vi "SDKSID4_Array Analysis.vi"(0 "SDKSID4 session In":T1, 1 "Interferogram in (ArrayI16)":i16[][](array[numeric]), 11 "error in (no error)":errorcluster) -> (4 "SDKSID4 session Out":T1, 6 "Intensity out":sgl[][](array[numeric]), 10 "Phase out":sgl[][](array[numeric]), 14 "Tilt information out":cluster{"X-tilt":sgl, "Y-tilt":sgl}, 15 "error out":errorcluster)   [LabVIEW 2013]
doc: "This VI analyses an input interferogram (a 2D Int16 representation array) . It outputs an intensity and a phase map (as double precision arrays), as well as an array containing X and Y tilts. This tilt is removed from the output phase."
uses:
  Refnum SDKSID4 session.ctl
  SDKSID4_AnalysisArraySize.ctl
  SID4_SDK.dll
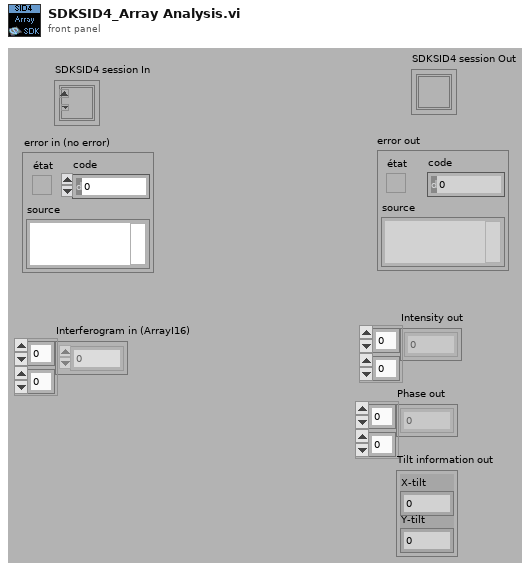
[diagram p1: front panel]
types:
  T1 = typedef "Refnum SDKSID4 session.ctl" = refnum<k1>
  T2 = typedef "SDKSID4_AnalysisArraySize.ctl" = cluster{"nRow":i32, "nCol":i32}
  T3 = typedef "SDKSID4_Analysis info.ctl" = cluster{"Grating position (mm)":dbl, "wavelength (nm)":dbl, "Remove background image":bool, "PhaseSize_width":i32, "PhaseSize_Height":i32}
  T4 = typedef "SDKSID4_ImageCameraSize.ctl" = cluster{"nRow":i32, "nCol":i32}
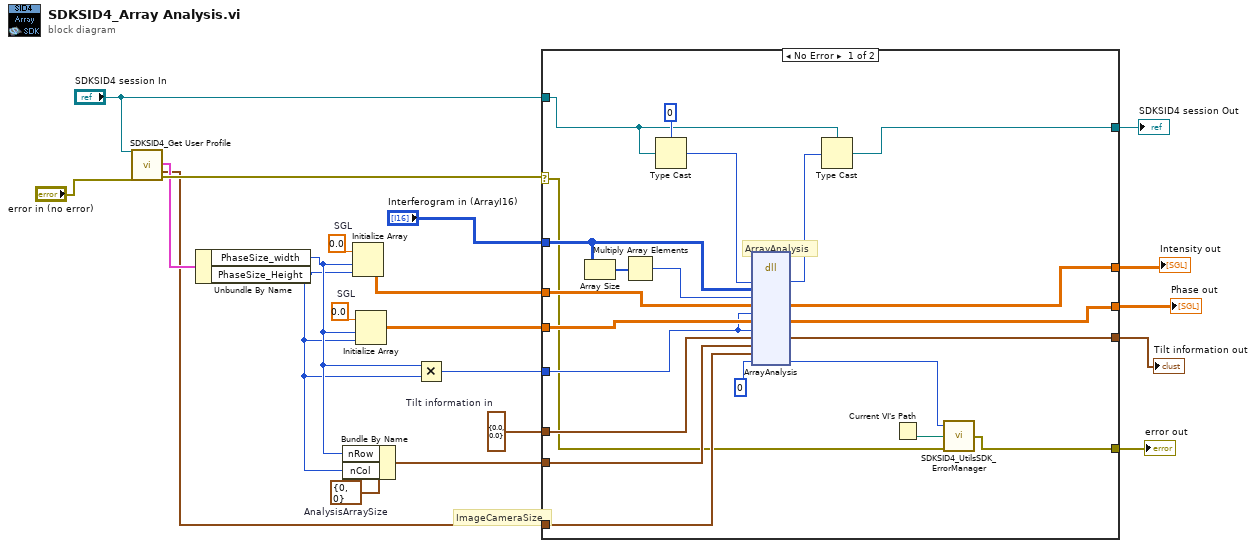
[diagram p0: block diagram]
diagram:
  w6 = sgl 0.0  # SGL
  w8 = T2 {"nRow"=0, "nCol"=0}  # AnalysisArraySize
  w14 = cluster{"X-tilt":sgl, "Y-tilt":sgl} {"X-tilt"=0.0, "Y-tilt"=0.0}  # Tilt information in
  w21 = sgl 0.0  # SGL
  # "ImageCameraSize"
  n1 = call "SDKSID4_Get User Profile.vi"("SDKSID4 session In"="SDKSID4 session In", "error in"="error in (no error)") -> ("Analysis info"=w9:T3, "ImageCameraSize"=w1:T4, "error out"=w19:errorcluster)  [unwired: 14 in, 9 out]
  n2 = Unbundle By Name(w9) -> ("PhaseSize_width"=w4:i32, "PhaseSize_Height"=w3:i32)
  n3 = Bundle By Name(cluster=w8, "nRow"=w4, "nCol"=w3) -> (w7:T2)
  n4 = Initialize Array(w21, w4, w3) -> (w16:sgl[][])
  n5 = Initialize Array(w6, w4, w3) -> (w5:sgl[][])
  n6 = Multiply(x=w4, y=w3) -> (x*y=w2:i32)
  n7 = case shown="No Error" w19 {
    selector: w19 -> [w24 w44]
    tunnel: "SDKSID4 session In" -> [w40 w47]
    tunnel: [w39 w47] -> w17
    tunnel: w16 -> [w34 w46]
    tunnel: "Interferogram in (ArrayI16)" -> [w31 _]
    tunnel: w14 -> [w35 w45]
    tunnel: [w28 w46] -> w13
    tunnel: [w27 w46] -> w12
    tunnel: [w26 w45] -> w11
    tunnel: [w23 w44] -> w10
    tunnel: w1 -> [w37 _]
    tunnel: w7 -> [w36 _]
    tunnel: w5 -> [w33 _]
    tunnel: w2 -> [w32 _]
    frame No Error {
      # "ArrayAnalysis"
      n8 = Array Size(array=w31) -> (size(s)=w30:i32[])
      n9 = Multiply Array Elements(1:w30) -> (0:w29:i32)
      n10 = Type Cast(type=u32 0, x=w40) -> (*(type *) &x=w42:u32)
      n11 = dll-call lib="C:/Program Files/SID4_SDK/DLL SDK/BIN/SID4_SDK.dll" fn="ArrayAnalysis"("SessionID"=w42, "InterferogramArrayI16"=w31, "interfero_bufSize"=w29, "Intensity"=w34, "intensity_bufSize"=w32, "Phase"=w33, "phase_bufSize"=w32, "Tilt information in"=w35, "AnalysisArraySize"=w36, "ImageCameraSize"=w37, "ErrorCode"=0) -> ("SessionID"=w41:i32, "Intensity"=w27:sgl[][], "Phase"=w28:sgl[][], "Tilt information in"=w26:cluster{"X-tilt":sgl, "Y-tilt":sgl}, "ErrorCode"=w22:i32)  [unwired: 10 in, 2 out]
      n12 = Type Cast(type=w40, x=w41) -> (*(type *) &x=w39:T1)
      n13 = Current VI's Path() -> (path=w25:path)
      n14 = call "SDKSID4_UtilsSDK_ErrorManager.vi"("error IN"=w24, "VI PathFile"=w25, "ErrorCode"=w22) -> ("error OUT"=w23:errorcluster)
    }
    frame Error {
    }
  }
  "error out" <- w10
  "SDKSID4 session Out" <- w17
  "Intensity out" <- w12
  "Phase out" <- w13
  "Tilt information out" <- w11
